vi "Configure Display.vi"(0 "VISA resource name":refnum<visa-resource-name>, 1 "Display (0: Normal)":u16(ring) items=["Normal", "Text", "Off"], 2 "Text (empty)":string, 5 "error in (no error)":errorcluster) -> (14 "VISA resource name out":refnum<visa-resource-name>, 19 "error out":errorcluster)   [LabVIEW 2016, in "Keithley 2000.lvlib"]
doc: "This VI configures the display of the instrument. It can turn the display on or off and also display custom text on the instrument."
uses:
  Keithley 2000.lvlib
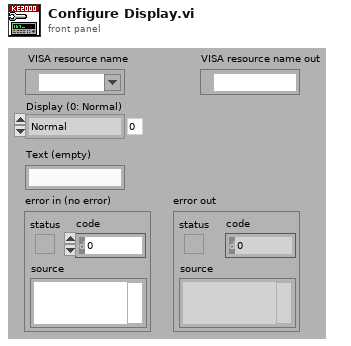
[diagram p1: front panel]
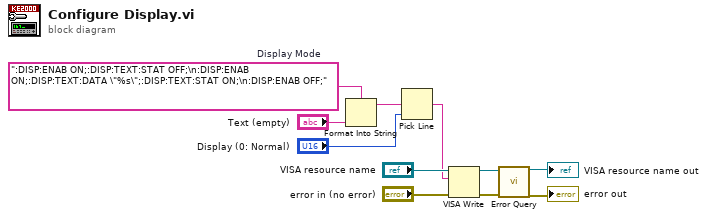
[diagram p0: block diagram]
diagram:
  w9 = ":DISP:ENAB ON;:DISP:TEXT:STAT OFF;\n:DISP:ENAB ON;:DISP:TEXT:DATA \"%s\";:DISP:TEXT:STAT ON;\n:DISP:ENAB OFF;"  # Display Mode
  n1 = Format Into String(format string=w9, "Text (empty)") -> (resulting string=w7:string)  [unwired: 2 in, 1 out]
  n2 = Pick Line(multi-line string=w7, line index="Display (0: Normal)") -> (output string=w5:string)  [unwired: 1 in]
  n3 = VISA Write(VISA resource name="VISA resource name", write buffer=w5, error in (no error)="error in (no error)") -> (VISA resource name out=w4:refnum<visa-resource-name>, error out=w3:errorcluster)  [unwired: 1 out]
  n4 = call "Error Query.vi"("VISA resource name"=w4, "error in (no error)"=w3) -> ("VISA resource name out"=→"VISA resource name out":refnum<visa-resource-name>, "error out"=→"error out":errorcluster)  [unwired: 14 in, 2 out]
